vi "Increment Filename.vi"(8 "error in (no error)":errorcluster, 11 "Path":path=path "C:/user/patrick/test/test/filename.itx") -> (0 "error out":errorcluster, 3 "Modified Path":path=path "C:/")   [LabVIEW 2016]
doc: "Given a <b>Path</b> ensure that it is not overwritten by appending a string of length 6.s\n\nExample:\nFilename.txt becomes Filename.000000.txt, where 000000 is automatically incremented to 000001 if 000000 already existis (et cetera)."
panel:
  out "Numeric":i32
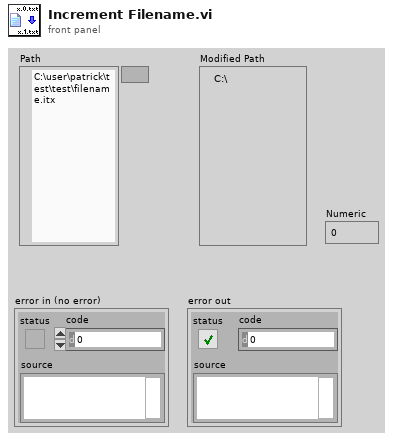
[diagram p1: front panel]
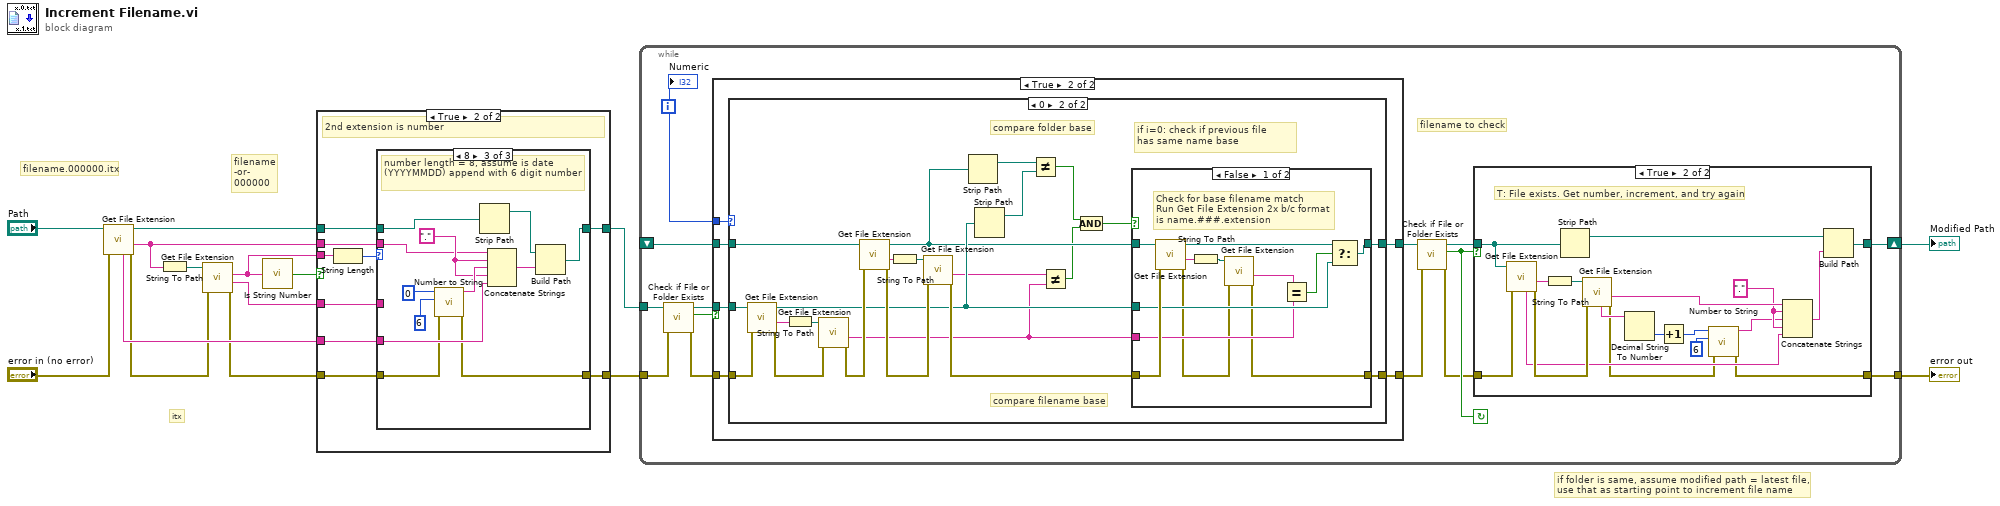
[diagram p0: block diagram]
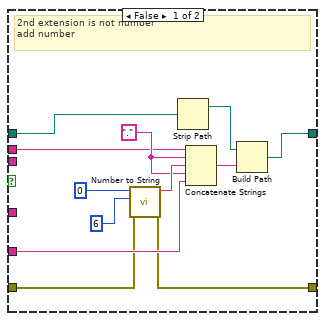
[diagram p2: hidden frame]
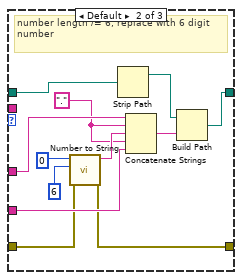
[diagram p4: hidden frame]
diagram:
  # "filename\n-or-\n000000"
  # "itx"
  # "filename.000000.itx"
  # "if folder is same, assume modified path = latest file,\nuse that as starting point to increment file name"
  n1 = call <vilib>:"Get File Extension.vi"("error in (no error)"="error in (no error)", "file"="Path") -> ("error out"=w7:errorcluster, "filename without extension"=w8:string, "dup file"=w5:path, "unmodified file extension"=w11:string)  [unwired: 6 out]
  n2 = String To Path(string=w8) -> (path=w9:path)
  n3 = call <vilib>:"Get File Extension.vi"("error in (no error)"=w7, "file"=w9) -> ("error out"=w6:errorcluster, "filename without extension"=w1:string, "lowercase file extension"=w2:string)  [unwired: 7 out]
  n4 = call "Is String Number.vi"("String"=w2) -> ("digit?"=w3:bool)
  n5 = case shown="True" w3 {
    tunnel: w11 -> [w26 w32]
    tunnel: [w21 w35] -> w10
    tunnel: w8 -> [w20 w28]
    tunnel: w6 -> [w19 w36]
    tunnel: w5 -> [w16 w34]
    tunnel: [w17 w33] -> w4
    tunnel: w2 -> [_ w31]
    tunnel: w1 -> [_ w29]
    frame False {
      w22 = "."
      # "2nd extension is not number\nadd number"
      n6 = call "Number to String.vi"("error in (no error)"=w19, "desired minimum string length"=6, "Number"=0 ("number")) -> ("error out"=w21:errorcluster, "String"=w23:string)  [unwired: 7 in]
      n7 = Strip Path(path=w16) -> (stripped path=w25:path)  [unwired: 1 out]
      n8 = Concatenate Strings(w20, w22, w23, w22, w26) -> (w27:string)
      n9 = Build Path(base path=w25, name or relative path=w27) -> (appended path=w17:path)
    }
    frame True {
      # "2nd extension is number"
      n10 = String Length(string=w31) -> (length=w30:i32)
      n11 = case shown="8" w30 {
        tunnel: w36 -> [w37 w40 w53]
        tunnel: [w37 w41 w54] -> w35
        tunnel: w34 -> [w38 w45 w57]
        tunnel: [w38 w44 w56] -> w33
        tunnel: w32 -> [_ w43 w55]
        tunnel: w29 -> [_ w42 _]
        tunnel: w28 -> [_ _ w51]
        frame 6 {
          # "number length is 6, do nothing"
        }
        frame Default {
          w39 = "."
          # "number length /= 6, replace with 6 digit number"
          n12 = call "Number to String.vi"("error in (no error)"=w40, "desired minimum string length"=6, "Number"=0 ("number")) -> ("error out"=w41:errorcluster, "String"=w47:string)  [unwired: 7 in]
          n13 = Strip Path(path=w45) -> (stripped path=w49:path)  [unwired: 1 out]
          n14 = Concatenate Strings(w42, w39, w47, w39, w43) -> (w50:string)
          n15 = Build Path(base path=w49, name or relative path=w50) -> (appended path=w44:path)
        }
        frame 8 {
          w52 = "."
          # "number length = 8, assume is date (YYYYMMDD) append with 6 digit number"
          n16 = call "Number to String.vi"("error in (no error)"=w53, "desired minimum string length"=6, "Number"=0 ("number")) -> ("error out"=w54:errorcluster, "String"=w59:string)  [unwired: 7 in]
          n17 = Strip Path(path=w57) -> (stripped path=w61:path)  [unwired: 1 out]
          n18 = Concatenate Strings(w51, w52, w59, w52, w55) -> (w62:string)
          n19 = Build Path(base path=w61, name or relative path=w62) -> (appended path=w56:path)
        }
      }
    }
  }
  n20 = while {
    shift-right: [w74] -> w14
    shift-left: _ -> [w69]
    tunnel: w10 -> [w65]
    tunnel: [w72] -> w12
    tunnel: w4 -> [w66]
    i -> [w68]
    stop <- w75 continue-if-true
    # "filename to check"
    n21 = call <vilib>:"Check if File or Folder Exists.vi"("error in (no error)"=w65, "path"=w66) -> ("error out"=w64:errorcluster, "file or folder exists?"=w63:bool, "dup path"=w67:path)  [unwired: 7 out]
    n22 = case shown="True" w63 {
      tunnel: [w78 w84] -> w71
      tunnel: [w77 w83] -> w70
      tunnel: w69 -> [_ w82]
      tunnel: w68 -> [_ w81]
      tunnel: w67 -> [w77 w80]
      tunnel: w64 -> [w78 w79]
      frame False {
        # "If file.000000.* doesn't exist, just skip this step"
      }
      frame True {
        n23 = case shown="0" w81 {
          tunnel: [w85 w108] -> w84
          tunnel: w80 -> [_ w102]
          tunnel: w79 -> [w85 w107]
          tunnel: [w86 w106] -> w83
          tunnel: w82 -> [w86 w99]
          frame Default {
            # "if i>0, you can't use previous file and you're going to have to scan through\nthe entire directory"
          }
          frame 0 {
            # "compare filename base"
            # "compare folder base"
            # "if i=0: check if previous file\nhas same name base"
            n24 = call <vilib>:"Get File Extension.vi"("error in (no error)"=w107, "file"=w102) -> ("error out"=w103:errorcluster, "filename without extension"=w104:string, "dup file"=w93:path)  [unwired: 7 out]
            n25 = String To Path(string=w104) -> (path=w105:path)
            n26 = call <vilib>:"Get File Extension.vi"("error in (no error)"=w103, "file"=w105) -> ("error out"=w96:errorcluster, "filename without extension"=w90:string)  [unwired: 8 out]
            n27 = call <vilib>:"Get File Extension.vi"("error in (no error)"=w96, "file"=w99) -> ("error out"=w94:errorcluster, "filename without extension"=w98:string, "dup file"=w92:path)  [unwired: 7 out]
            n28 = String To Path(string=w98) -> (path=w97:path)
            n29 = call <vilib>:"Get File Extension.vi"("error in (no error)"=w94, "file"=w97) -> ("error out"=w95:errorcluster, "filename without extension"=w91:string)  [unwired: 8 out]
            n30 = Strip Path(path=w92) -> (stripped path=w100:path)  [unwired: 1 out]
            n31 = Strip Path(path=w93) -> (stripped path=w101:path)  [unwired: 1 out]
            n32 = Not Equal?(x=w100, y=w101) -> (x != y?=w87:bool)
            n33 = Not Equal?(x=w91, y=w90) -> (x != y?=w89:bool)
            n34 = And(x=w87, y=w89) -> (x .and. y?=w88:bool)
            n35 = case shown="False" w88 {
              tunnel: [w110 w121] -> w108
              tunnel: w90 -> [w114 _]
              tunnel: w95 -> [w120 w121]
              tunnel: w93 -> [w117 w122]
              tunnel: w92 -> [w116 _]
              tunnel: [w115 w122] -> w106
              frame False {
                # "Check for base filename match\nRun Get File Extension 2x b/c format\nis name.###.extension"
                n36 = call <vilib>:"Get File Extension.vi"("error in (no error)"=w120, "file"=w116) -> ("error out"=w111:errorcluster, "filename without extension"=w112:string, "dup file"=w119:path)  [unwired: 7 out]
                n37 = String To Path(string=w112) -> (path=w113:path)
                n38 = call <vilib>:"Get File Extension.vi"("error in (no error)"=w111, "file"=w113) -> ("error out"=w110:errorcluster, "filename without extension"=w109:string)  [unwired: 8 out]
                n39 = Equal?(x=w109, y=w114) -> (x = y?=w118:bool)
                n40 = Select(t=w119, s=w118, f=w117) -> (s? t:f=w115:path)
              }
              frame True {
                # "If no previous file use new one"
              }
            }
          }
        }
      }
    }
    n41 = call <vilib>:"Check if File or Folder Exists.vi"("error in (no error)"=w71, "path"=w70) -> ("error out"=w73:errorcluster, "file or folder exists?"=w75:bool, "dup path"=w76:path)  [unwired: 7 out]
    n42 = case shown="True" w75 {
      tunnel: w76 -> [w124 w142]
      tunnel: [w124 w141] -> w74
      tunnel: w73 -> [w123 w133]
      tunnel: [w123 w126] -> w72
      frame False {
        # "F: file doesn't exist. Exit"
      }
      frame True {
        w137 = "." ("regular expression")
        # "T: File exists. Get number, increment, and try again"
        n43 = call <vilib>:"Get File Extension.vi"("error in (no error)"=w133, "file"=w142) -> ("error out"=w132:errorcluster, "filename without extension"=w131:string, "unmodified file extension"=w130:string)  [unwired: 7 out]
        n44 = String To Path(string=w131) -> (path=w139:path)
        n45 = Strip Path(path=w142) -> (stripped path=w134:path)  [unwired: 1 out]
        n46 = call <vilib>:"Get File Extension.vi"("error in (no error)"=w132, "file"=w139) -> ("error out"=w127:errorcluster, "filename without extension"=w138:string, "unmodified file extension"=w129:string)  [unwired: 7 out]
        n47 = Decimal String To Number(string=w129) -> (number=w135:i32)  [unwired: 1 in, 2 out]
        n48 = Increment(x=w135) -> (x+1=w136:i32)
        n49 = call "Number to String.vi"("error in (no error)"=w127, "desired minimum string length"=6, "Number"=w136) -> ("error out"=w126:errorcluster, "String"=w128:string)  [unwired: 7 in]
        n50 = Concatenate Strings(w138, w137, w128, w137, w130) -> (w140:string)
        n51 = Build Path(base path=w134, name or relative path=w140) -> (appended path=w141:path)
      }
    }
    "Numeric" <- w68
  }
  "Modified Path" <- w14
  "error out" <- w12
